vi "CRYCurve Library.vi"() -> ()   [LabVIEW 2013]
uses:
  <vilib>/Utility/miscctls.llb/LVPoint32TypeDef.ctl
  <vilib>/Utility/miscctls.llb/LVBoundsTypeDef.ctl
  <vilib>/Utility/inputDevices.llb/closeMouse.vi
  Global/CRYCurve Library Global.vi
  <vilib>/Utility/inputDevices.llb/mouseAcquire.vi
panel:
  out "StepNameChange":i32
  in  "DragStartFlag":bool
  out "Drop?":bool
  out "AllDragTags":string[](array[string])
  in  "GroupFlag":bool
  out "AllParents":string[](array[string])
  out "Select Row":i32
  out "GroupRowNumber":i32
  out "TreeValue":string[](array[string])
  out "Menu Coords":T1
  in  "Legend":i32(listbox)
  out "OldPos":T2
  out "Coords":T1
  in  "StateOut":bool
  in  "stop":bool
  in  "UndoAutoProtect":bool
  in  "AutoProtect":bool
  in  "CompleteDelete":bool
  in  "Protect":bool
  in  "Delete":bool
  in  "Save":bool
  in  "Open":bool
  out "BottomBar":bool
  in  "CurveLibrary Tab":enum32{"Curves", "Values", "Results", "WFM"}(tab)
  in  "Curves Tree":string[](tree)
  in  "Values Tree":string[](tree)
  in  "Results Tree":string[](tree)
  in  "WFM Tree":string[](tree)
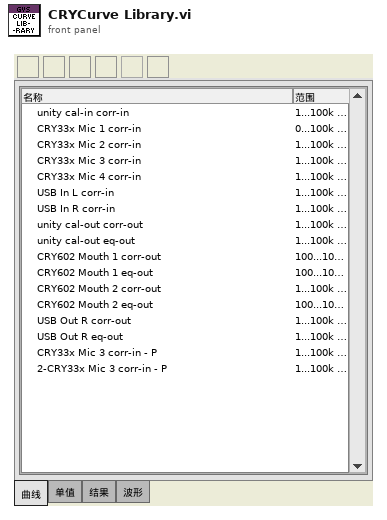
[diagram p1: front panel]
types:
  T1 = typedef "LVPoint32TypeDef.ctl" = cluster{"Horizontal":i32, "Vertical":i32}
  T2 = typedef "LVBoundsTypeDef.ctl" = cluster{"Width":u32, "Height":u32}
  T3 = typedef "CRYCurveLib Info Cluster.ctl" = cluster{"GroupingState":string}
  T4 = cluster{"Horizontal":i32, "Vertical":i32, "Scrolling":i32}
  T5 = cluster{"Shift":bool, "Ctrl":bool, "Alt":bool, "Cmd":bool, "Opt":bool}
  T6 = cluster{"data name":string, "drag data":variant}[]
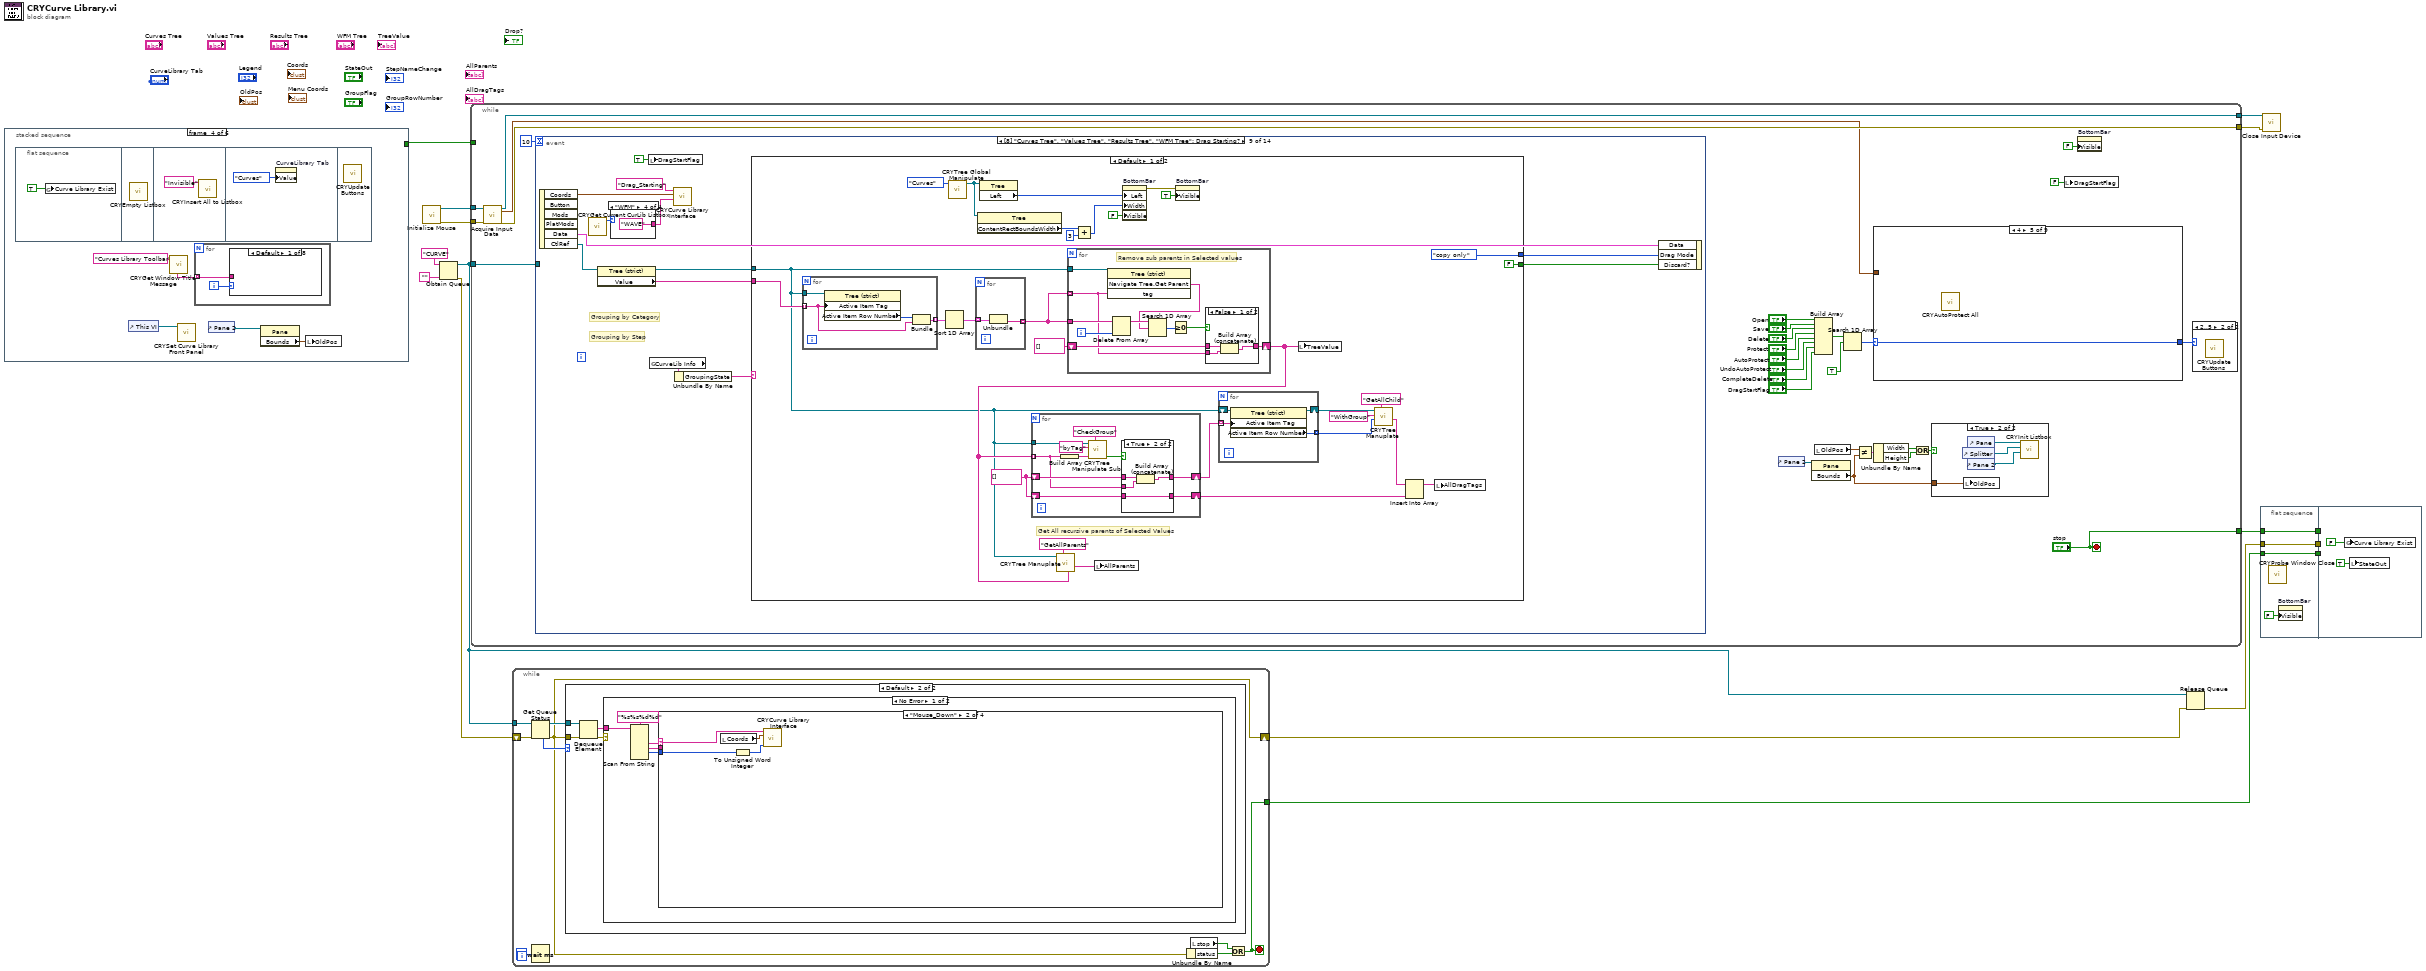
[diagram p0: block diagram]
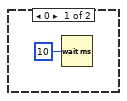
[diagram p2: hidden frame]
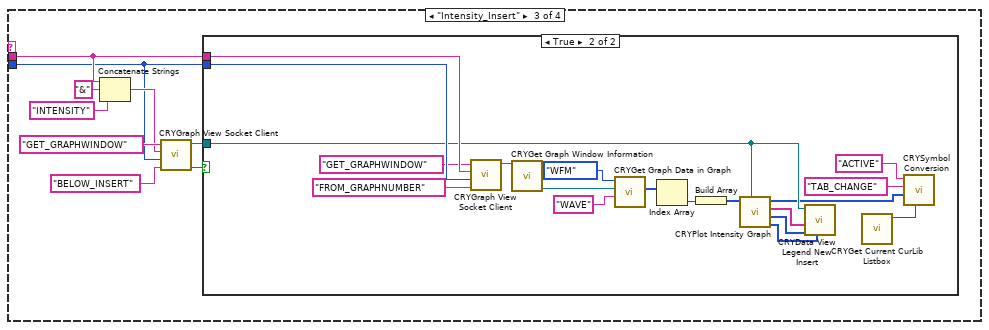
[diagram p4: hidden frame]
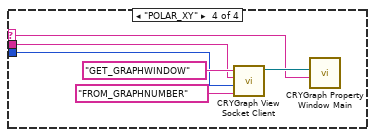
[diagram p6: hidden frame]
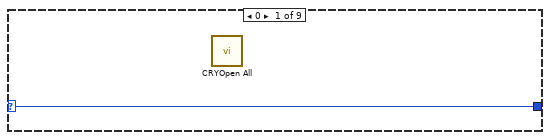
[diagram p10: hidden frame]
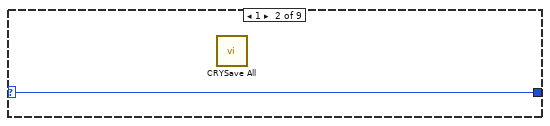
[diagram p11: hidden frame]
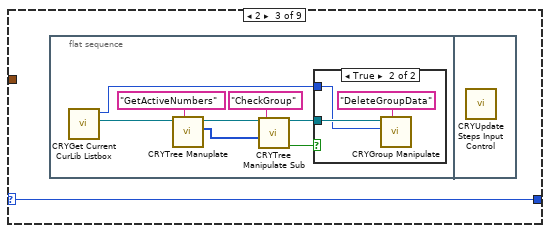
[diagram p12: hidden frame]
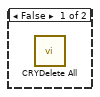
[diagram p13: hidden frame]
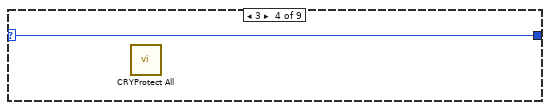
[diagram p14: hidden frame]
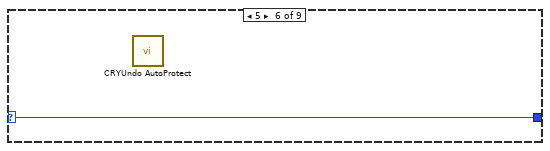
[diagram p15: hidden frame]
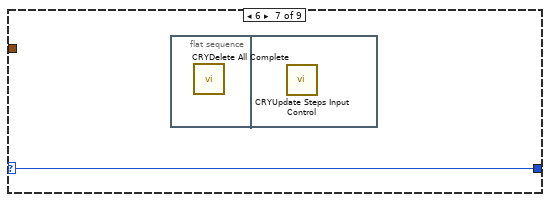
[diagram p16: hidden frame]
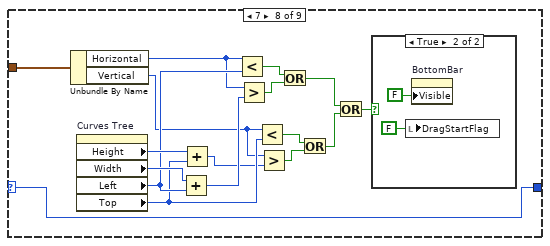
[diagram p17: hidden frame]
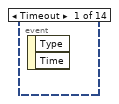
[diagram p20: hidden frame]
diagram:
  n1 = stacked-sequence {
    tunnel: [_ _ _ _ _ w68] -> w13
    frame #0 {
      n2 = control-ref of="Curves Tree"() -> (w19:refnum<vi>)
      n3 = control-ref of="Values Tree"() -> (w18:refnum<vi>)
      n4 = control-ref of="Results Tree"() -> (w17:refnum<vi>)
      n5 = control-ref of="WFM Tree"() -> (w28:refnum<vi>)
      n6 = control-ref of="CurveLibrary Tab"() -> (w27:refnum<vi>)
      n7 = control-ref of="Open"() -> (w26:refnum<vi>)
      n8 = control-ref of="Save"() -> (w25:refnum<vi>)
      n9 = control-ref of="Delete"() -> (w24:refnum<vi>)
      n10 = control-ref of="Protect"() -> (w23:refnum<vi>)
      n11 = control-ref of="AutoProtect"() -> (w22:refnum<vi>)
      n12 = control-ref of="UndoAutoProtect"() -> (w21:refnum<vi>)
      n13 = control-ref of="This VI"() -> (w20:refnum<vi>)
      n14 = global write "CRYCurve Library Global.vi" "Curve Library VI"(w20) -> ()
      n15 = global write "CRYCurve Library Global.vi" "Curves Tree"(w19) -> ()
      n16 = global write "CRYCurve Library Global.vi" "Values Tree"(w18) -> ()
      n17 = global write "CRYCurve Library Global.vi" "Results Tree"(w17) -> ()
      n18 = global write "CRYCurve Library Global.vi" "WFM Tree"(w28) -> ()
      n19 = global write "CRYCurve Library Global.vi" "Curve Library Tab"(w27) -> ()
      n20 = global write "CRYCurve Library Global.vi" "Open Button"(w26) -> ()
      n21 = global write "CRYCurve Library Global.vi" "Save Button"(w25) -> ()
      n22 = global write "CRYCurve Library Global.vi" "Delete Button"(w24) -> ()
      n23 = global write "CRYCurve Library Global.vi" "Protect Button"(w23) -> ()
      n24 = global write "CRYCurve Library Global.vi" "AutoProtect Button"(w22) -> ()
      n25 = global write "CRYCurve Library Global.vi" "UndoAutoProtect Button"(w21) -> ()
      n26 = local write "stop"(FALSE ("stop")) -> ()
    }
    frame #1 {
      n27 = while {
        tunnel: [w31] -> w30
        stop <- w31 stop-if-true
        n28 = global read "CRYCurve Library Global.vi" "Curve Library Global Inserting"() -> (w32:bool)
        n29 = Wait Until Next ms Multiple(millisecond multiple=u32 10 ("milliseconds to wait")) -> ()  [unwired: 1 out]
        n30 = Not(x=w32) -> (.not. x?=w31:bool)
      }
      n31 = global write "CRYCurve Library Global.vi" "Curve Library Loading"(w30) -> ()
    }
    frame #2 {
      n32 = control-ref of="Splitter"() -> (w35:refnum<vi>)
      n33 = control-ref of="Pane"() -> (w36:refnum<vi>)
      n34 = control-ref of="Pane 2"() -> (w34:refnum<vi>)
      n35 = call "CRYInit Listbox.vi"("Pane 2"=w34, "Splitter"=w35, "Pane 1"=w36) -> ()  [unwired: 9 out]
    }
    frame #3 {
      n36 = flat-sequence {
        frame #0 {
          n37 = global write "CRYCurve Library Global.vi" "Curve Library Exist"(TRUE ("Exist")) -> ()
        }
        frame #1 {
          n38 = call "CRYEmpty Listbox.vi"() -> ()  [unwired: 1 out]
        }
        frame #2 {
          n39 = call "CRYInsert All to Listbox.vi"("sAction"="Invisible") -> ()  [unwired: 11 out]
        }
        frame #3 {
          n40 = property on="CurveLibrary Tab" class="TabCtl (strict)"("Value"=enum32{"Curves", "Values", "Results", "WFM"}."Curves" ("Curve Library Tab")) -> ()  [unwired: 2 in, 2 out]
        }
        frame #4 {
          n41 = call "CRYUpdate Buttons.vi"() -> ()  [unwired: 1 in, 11 out]
        }
      }
      n42 = control-ref of="This VI"() -> (w37:refnum<vi>)
      n43 = call "CRYGet Window Title Message.vi"("Kind"="Curves Library Toolbar") -> ("Tip Strip"=w40:string[])  [unwired: 5 in, 5 out]
      n44 = call "CRYSet Curve Library Front Panel.vi"("Vi Ref In"=w37) -> ()  [unwired: 10 in, 1 out]
      n45 = for {
        tunnel: w40 -> [w42] mode=indexing
        i -> [w43]
        n46 = case shown="Default" w43 {
          tunnel: w42 -> [_ w44 w45 w46 w47 w48 w49 w50]
          frame Default {
          }
          frame 0 {
            n47 = property on="Open" class="Bool"("TipStrip"=w44) -> ()  [unwired: 2 in, 2 out]
          }
          frame 1 {
            n48 = property on="Save" class="Bool"("TipStrip"=w45) -> ()  [unwired: 2 in, 2 out]
          }
          frame 2 {
            n49 = property on="Delete" class="Bool"("TipStrip"=w46) -> ()  [unwired: 2 in, 2 out]
          }
          frame 3 {
            n50 = property on="Protect" class="Bool"("TipStrip"=w47) -> ()  [unwired: 2 in, 2 out]
          }
          frame 4 {
            n51 = property on="AutoProtect" class="Bool"("TipStrip"=w48) -> ()  [unwired: 2 in, 2 out]
          }
          frame 5 {
            n52 = property on="UndoAutoProtect" class="Bool"("TipStrip"=w49) -> ()  [unwired: 2 in, 2 out]
          }
          frame 6 {
            n53 = property on="CompleteDelete" class="Bool"("TipStrip"=w50) -> ()  [unwired: 2 in, 2 out]
          }
        }
      }
      n54 = control-ref of="Pane 2"() -> (w38:refnum<vi>)
      n55 = property class="Pane"(reference=w38) -> ("Bounds"=w39:T2)  [unwired: 1 in, 2 out]
      n56 = local write "OldPos"(w39) -> ()
    }
    frame #4 {
      n57 = flat-sequence {
        frame #0 {
          n58 = call "CRYGroup Manipulate.vi"("sAction"="GroupingOff", "sOption"="Invisible") -> ()  [unwired: 6 in, 4 out]
        }
        frame #1 {
          n59 = global read "CRYCurve Library Global.vi" "CurveLib Info"() -> (w57:T3)
          n60 = Unbundle By Name(w57) -> ("GroupingState"=w56:string)
          n61 = case shown="\"Grouping by Category\"" w56 {
            frame "Grouping Off", Default {
              n62 = call "CRYTree Global Manipulate.vi"("sOption"="All") -> ("WFM Tree"=w59:refnum<vi>, "Results Tree"=w60:refnum<vi>, "Values Tree"=w61:refnum<vi>, "Tree/Curve Tree"=w62:refnum<vi>)  [unwired: 7 in]
              n63 = Build Array(w62, w61, w60, w59) -> (w58:refnum<vi>[])
              n64 = for {
                tunnel: w58 -> [w65] mode=indexing
                n65 = property class="Tree"(reference=w65, "Visible"=TRUE) -> ()  [unwired: 1 in, 2 out]
              }
            }
            frame "Grouping by Category" {
              n66 = call "CRYGroup Manipulate.vi"("sAction"="GroupingbyCategory") -> ()  [unwired: 7 in, 4 out]
            }
            frame "Grouping by Step" {
              n67 = call "CRYGroup Manipulate.vi"("sAction"="GroupingbyStep") -> ()  [unwired: 7 in, 4 out]
            }
          }
        }
      }
    }
    frame #5 {
      w68 = FALSE ("Curve Library Loading")
      n68 = call "CRYTree Global Manipulate.vi"("Type In"=enum16{"Curves", "Values", "Results", "WFM"}."Curves") -> ("Tree/Curve Tree"=w73:refnum<vi>)  [unwired: 7 in, 3 out]
      n69 = property class="Tree"(reference=w73) -> ("ContentRectBoundsWidth"=w70:i32)  [unwired: 1 in, 2 out]
      n70 = property class="Tree"(reference=w73) -> ("Left"=w76:i32)  [unwired: 1 in, 2 out]
      n71 = global write "CRYCurve Library Global.vi" "Curve Library Loading"(w68) -> ()
      n72 = local write "DragStartFlag"(w68) -> ()
      n73 = local write "GroupRowNumber"(-1 ("GroupRowNumber")) -> ()
      n74 = Add(x=w70, y=3) -> (x+y=w69:i32)
      n75 = local write "StateOut"(TRUE ("StateOut")) -> ()
      n76 = property on="BottomBar" class="Bool (strict)"("Left"=w76, "Width"=w69, "Visible"=FALSE) -> ()  [unwired: 2 in, 2 out]
    }
  }
  n77 = call <vilib>:"Initialize Mouse.vi"() -> ("error out"=w3:errorcluster, "device ID"=w4:refnum<k1>)  [unwired: 10 in]
  n78 = Obtain Queue(name (unnamed)="CURVE" ("YAxisTitle"), element data type="" ("Action Type")) -> (queue out=w7:refnum<queue>, error out=w6:errorcluster)  [unwired: 3 in, 1 out]
  n79 = while {
    tunnel: w13 -> [_]
    tunnel: ["stop"] -> w12
    tunnel: w7 -> [w101]
    tunnel: w4 -> [w88]
    tunnel: w3 -> [w87]
    tunnel: [w86] -> w2
    tunnel: [w85] -> w1
    stop <- "stop" stop-if-true
    n80 = call-poly <vilib>:"Acquire Input Data.vi"("device ID"=w88, "error in (no error)"=w87) -> ("device ID"=w86:refnum<k1>, "axis info"=w82:T4, "error out"=w85:errorcluster)  [unwired: 14 in, 1 out]
    n81 = event shown="[8] \"Curves Tree\", \"Values Tree\", \"Results Tree\", \"WFM Tree\": Drag Starting?" {
      selector: _ -> [_ _ _ _ _ _ _ _ _ _ _ _ _ _]
      dyn-events: _ -> [_ _ _ _ _ _ _ _ _ _ _ _ _ _]
      timeout: 10 -> [_ _ _ _ _ _ _ _ _ _ _ _ _ _]
      tunnel: w101 -> [_ _ _ _ _ w170 _ _ _ _ _ _ _ _]
      event Timeout {
        n82 = event-data() -> ()  [unwired: 3 out]
      }
      event "CurveLibrary Tab": Value Change {
        n83 = event-data() -> ("NewVal"=w150:enum32{"Curves", "Values", "Results", "WFM"})  [unwired: 6 out]
        n84 = local write "GroupRowNumber"(-1 ("GroupRowNumber")) -> ()
        n85 = call "CRYCurve Library Interface.vi"("nButton"=w150, "sEventName"="Tab_Value_Change") -> ()  [unwired: 9 in, 1 out]
      }
      event Pane Size {
        n86 = event-data() -> ()  [unwired: 7 out]
        n87 = control-ref of="Splitter"() -> (w153:refnum<vi>)
        n88 = call "CRYTree Global Manipulate.vi"("Type In"=enum16{"Curves", "Values", "Results", "WFM"}."Curves") -> ("Tree/Curve Tree"=w159:refnum<vi>)  [unwired: 7 in, 3 out]
        n89 = control-ref of="Pane"() -> (w154:refnum<vi>)
        n90 = control-ref of="Pane 2"() -> (w152:refnum<vi>)
        n91 = property class="Tree"(reference=w159) -> ("ContentRectBoundsWidth"=w155:i32)  [unwired: 1 in, 2 out]
        n92 = call "CRYInit Listbox.vi"("Pane 2"=w152, "Splitter"=w153, "Pane 1"=w154) -> ()  [unwired: 9 in]
        n93 = Add(x=w155, y=3) -> (x+y=w157:i32)
        n94 = property on="BottomBar" class="Bool (strict)"("Width"=w157) -> ()  [unwired: 2 in, 2 out]
      }
      event "Curves Tree", "Values Tree", "Results Tree", "WFM Tree": Shortcut Menu Activation? {
        n95 = event-data() -> ("MenuRef"=w162:refnum<k9>, "Coords"=w161:T1)  [unwired: 1 out]
        n96 = local write "Menu Coords"(w161) -> ()
        n97 = call "CRYCurve Library Interface.vi"("MenuRef"=w162, "Coords"=w161, "sEventName"="Shortcut_Menu_Activation") -> ("bResult"=w160:bool)  [unwired: 8 in]
        n98 = event-data("Discard?"=w160) -> ()  [unwired: 1 in, 1 out]
      }
      event "Curves Tree", "Values Tree", "Results Tree", "WFM Tree": Shortcut Menu Selection (User) {
        n99 = event-data() -> ("ItemTag"=w165:string)  [unwired: 2 out]
        n100 = local read "Menu Coords"() -> (w164:T1)
        n101 = call "CRYCurve Library Interface.vi"("sData"=w165, "Coords"=w164, "sEventName"="Shortcut_Menu_Selection") -> ()  [unwired: 8 in, 1 out]
      }
      event "Curves Tree", "Values Tree", "Results Tree", "WFM Tree": Mouse Down {
        n102 = event-data() -> ("Coords"=w169:T1, "Button"=w168:u16)  [unwired: 2 out]
        n103 = flat-sequence {
          tunnel: w169 -> [w172]
          tunnel: w168 -> [w173]
          tunnel: [w173] -> w171
          tunnel: [w172] -> w167
          tunnel: w171 -> [w177]
          tunnel: w170 -> [_]
          tunnel: w167 -> [w176]
          frame #0 {
            n104 = To Unsigned Word Integer(number=w173) -> (unsigned 16bit integer=w175:u16)
            n105 = call "CRYCurve Library Interface.vi"("nButton"=w175, "Coords"=w172, "sEventName"="Mouse_Down_Right") -> ()  [unwired: 8 in, 1 out]
          }
          frame #1 {
            n106 = call "CRYCurve Library Interface.vi"("nButton"=w177, "Coords"=w176, "sEventName"="Mouse_Down") -> ()  [unwired: 8 in, 1 out]
          }
        }
      }
      event "Curves Tree", "Values Tree", "Results Tree", "WFM Tree": Key Down {
        n107 = event-data() -> ("ScanCode"=w180:i16, "PlatMods"=w179:T5)  [unwired: 2 out]
        n108 = call "CRYCurve Library Interface.vi"("PlatMods"=w179, "nButton"=w180, "sEventName"="Key_Down") -> ()  [unwired: 8 in, 1 out]
      }
      event "Curves Tree", "Values Tree", "Results Tree", "WFM Tree": Double Click {
        n109 = event-data() -> ("Coords"=w182:T1)  [unwired: 5 out]
        n110 = call "CRYCurve Library Interface.vi"("Coords"=w182, "sEventName"="Double_Click") -> ()  [unwired: 9 in, 1 out]
      }
      event "Curves Tree", "Values Tree", "Results Tree", "WFM Tree": Drag Starting? {
        # "Grouping by Step"
        # "Grouping by Category"
        n111 = event-data() -> ("Coords"=w195:T1, "Data"=w191:T6, "CtlRef"=w190:refnum<vi>)  [unwired: 4 out]
        n112 = call "CRYGet Current CurLib Listbox.vi"() -> ("Type"=w193:enum16{"Curves", "Values", "Results", "WFM"})  [unwired: 9 in, 2 out]
        n113 = property class="Tree (strict)"(reference=w190) -> (reference out=w188:refnum<vi>, "Value"=w189:string[])  [unwired: 1 in, 1 out]
        n114 = case shown="\"WFM\"" w193 {
          tunnel: ["XY" ("GraphType") "TABLE" ("GraphType") "RESULT" ("GraphType") "WAVE" ("GraphType")] -> w192
          frame "Curves", Default {
          }
          frame "Values" {
          }
          frame "Results" {
          }
          frame "WFM" {
          }
        }
        n115 = local write "DragStartFlag"(TRUE ("DragStartFlag")) -> ()
        n116 = global read "CRYCurve Library Global.vi" "CurveLib Info"() -> (w186:T3)
        n117 = call "CRYCurve Library Interface.vi"("sData"=w192, "Coords"=w195, "sEventName"="Drag_Starting") -> ()  [unwired: 8 in, 1 out]
        n118 = Unbundle By Name(w186) -> ("GroupingState"=w185:string)
        n119 = case shown="Default" w185 {
          tunnel: [enum32{"copy or move", "copy only", "move only"}."copy only" ("Drag Mode") enum32{"copy or move", "copy only", "move only"}."copy only" ("Drag Mode")] -> w196
          tunnel: w189 -> [w223 _]
          tunnel: w188 -> [w211 _]
          tunnel: [FALSE ("Discard?") TRUE ("Discard?")] -> w184
          frame Default {
            w215 = string[] []
            # "Get All recursive parents of Selected Values"
            n120 = for {
              tunnel: w223 -> [w265] mode=indexing
              tunnel: w211 -> [w267]
              tunnel: [w264] -> w222 mode=indexing
              n121 = property class="Tree (strict)"(reference=w267, "Active Item Tag"=w265) -> ("Active Item Row Number"=w266:i32)  [unwired: 1 in, 2 out]
              n122 = Bundle("Active Item Row Number"=w266, w265) -> (w264:cluster{"Active Item Row Number":i32, string})  [unwired: 1 in]
            }
            n123 = Sort 1D Array(array=w222) -> (sorted array=w221:cluster{"Active Item Row Number":i32, string}[])
            n124 = call "CRYTree Global Manipulate.vi"("Type In"=enum16{"Curves", "Values", "Results", "WFM"}."Curves") -> ("Tree/Curve Tree"=w201:refnum<vi>)  [unwired: 7 in, 3 out]
            n125 = for {
              tunnel: w221 -> [w263] mode=indexing
              tunnel: [w262] -> w220 mode=indexing
              n126 = Unbundle(w263) -> (w262:string)  [unwired: 1 out]
            }
            n127 = property class="Tree"(reference=w201) -> ("ContentRectBoundsWidth"=w204:i32)  [unwired: 1 in, 2 out]
            n128 = property class="Tree"(reference=w201) -> ("Left"=w199:i32)  [unwired: 1 in, 2 out]
            n129 = for {
              tunnel: w220 -> [w248] mode=indexing
              tunnel: w211 -> [w257]
              tunnel: w220 -> [w251]
              shift-right: [w253] -> w217
              shift-left: string[] [] -> [w254]
              i -> [w252]
              # "Remove sub parents in Selected values"
              n130 = invoke class="Tree (strict)" method="Navigate Tree.Get Parent"(reference=w257, "tag"=w248) -> ("Navigate Tree:Get Parent"=w249:string)  [unwired: 2 in, 3 out]
              n131 = Delete From Array(array=w251, index=w252) -> (array with subset deleted=w250:string[])  [unwired: 1 in, 1 out]
              n132 = Search 1D Array(1D array=w250, element=w249) -> (index of element=w256:i32)  [unwired: 1 in]
              n133 = Greater Or Equal To 0?(x=w256) -> (x >= 0?=w255:bool)
              n134 = case shown="False" w255 {
                tunnel: w254 -> [w260 w261]
                tunnel: [w259 w261] -> w253
                tunnel: w248 -> [w258 _]
                frame False {
                  n135 = Build Array (concatenate)(w260, w258) -> (w259:string[])
                }
                frame True {
                }
              }
            }
            n136 = for {
              tunnel: w217 -> [w232] mode=indexing
              tunnel: w211 -> [w235]
              shift-right: [w239] -> w206
              shift-left: w215 -> [w238]
              shift-right: [w230] -> w214
              shift-left: w215 -> [w231]
              n137 = Build Array(w232) -> (w234:string[])
              n138 = call "CRYTree Manipulate Sub.vi"("sAction"="CheckGroup", "sData"=w234, "sOption"="byTag", "Tree in"=w235) -> ("bData out"=w233:bool)  [unwired: 3 in, 4 out]
              n139 = case shown="True" w233 {
                tunnel: w238 -> [w243 w247]
                tunnel: [w243 w246] -> w239
                tunnel: w232 -> [w241 w245]
                tunnel: w231 -> [w242 w244]
                tunnel: [w240 w244] -> w230
                frame False {
                  n140 = Build Array (concatenate)(w242, w241) -> (w240:string[])
                }
                frame True {
                  n141 = Build Array (concatenate)(w247, w245) -> (w246:string[])
                }
              }
            }
            n142 = call "CRYTree Manuplate.vi"("sData"=w217, "sAction"="GetAllParents", "Tree in"=w211) -> ("sData Out"=w216:string[])  [unwired: 5 in, 3 out]
            n143 = Add(x=w204, y=3) -> (x+y=w205:i32)
            n144 = local write "AllParents"(w216) -> ()
            n145 = property on="BottomBar" class="Bool (strict)"("Left"=w199, "Width"=w205, "Visible"=FALSE) -> (error out=w198:errorcluster)  [unwired: 2 in, 1 out]
            n146 = property on="BottomBar" class="Bool (strict)"(error in=w198, "Visible"=TRUE) -> ()  [unwired: 1 in, 2 out]
            n147 = for {
              tunnel: w206 -> [w228] mode=indexing
              tunnel: [w227] -> w209 mode=indexing
              shift-right: [w226] -> w210
              shift-left: w211 -> [w229]
              n148 = property class="Tree (strict)"(reference=w229, "Active Item Tag"=w228) -> (reference out=w226:refnum<vi>, "Active Item Row Number"=w227:i32)  [unwired: 1 in, 1 out]
            }
            n149 = local write "TreeValue"(w217) -> ()
            n150 = call "CRYTree Manuplate.vi"("sAction"="GetAllChild", "nData"=w209, "sOption"="WithGroup", "Tree in"=w210) -> ("sData Out"=w208:string[])  [unwired: 4 in, 3 out]
            n151 = Insert Into Array(array=w208, new element=w214) -> (w213:string[])  [unwired: 1 in]
            n152 = local write "AllDragTags"(w213) -> ()
          }
          frame "Grouping by Category", "Grouping by Step" {
          }
        }
        n153 = event-data("Data"=w191, "Drag Mode"=w196, "Discard?"=w184) -> ()  [unwired: 1 in, 1 out]
      }
      event "Curves Tree", "Values Tree", "Results Tree", "WFM Tree": event type 3.0.xa000003a {
        n154 = event-data() -> ("CtlRef"=w281:refnum<vi>, "Coords"=w309:T1)  [unwired: 8 out]
        n155 = Unbundle By Name(w309) -> ("Horizontal"=w293:i32, "Vertical"=w318:i32)
        n156 = local read "TreeValue"() -> (w280:string[])
        n157 = local read "AllDragTags"() -> (w279:string[])
        n158 = call "CRYGet Tree Click State.vi"("Coords"=w309, "Tree Ref In"=w281) -> ("Row Number"=w306:i32, "Tag"=w275:string)  [unwired: 4 in, 4 out]
        n159 = for {
          tunnel: w281 -> [w411]
          tunnel: w280 -> [w410] mode=indexing
          tunnel: [w409] -> w334 mode=indexing
          n160 = property class="Tree (strict)"(reference=w411, "Active Item Tag"=w410) -> ("Active Item Row Number"=w409:i32)  [unwired: 1 in, 2 out]
        }
        n161 = case shown="0, Default" w306 {
          selector: w306 -> [w374 _]
          tunnel: w281 -> [w378 w380]
          tunnel: [w376 w380] -> w308
          tunnel: [w375 FALSE ("bData out")] -> w327
          frame 0, Default {
            n162 = Build Array(w374) -> (w377:i32[])
            n163 = call "CRYTree Manipulate Sub.vi"("sAction"="CheckGroup", "nData"=w377, "Tree in"=w378) -> ("bData out"=w375:bool, "Tree Out"=w376:refnum<vi>)  [unwired: 4 in, 3 out]
          }
          frame -1 {
          }
        }
        n164 = case shown="True" w327 {
          tunnel: w318 -> [w389 w398]
          tunnel: w281 -> [w385 w406]
          tunnel: w306 -> [w384 w395]
          tunnel: [w383 w393] -> w311
          tunnel: [FALSE w396] -> w326
          frame False {
            n165 = Decrement(x=w384) -> (x-1=w387:i32)
            n166 = property class="Tree (strict)"(reference=w385, "Active Item Row Number"=w384, "ActiveColNum"=0 ("Active Cell:Active Column Number")) -> ("ActiveCellPosTop"=w388:i32)  [unwired: 1 in, 2 out]
            n167 = Add(x=w388, y=6) -> (x+y=w390:i32)
            n168 = Greater Or Equal?(x=w390, y=w389) -> (x >= y?=w386:bool)
            n169 = Select(t=w387, s=w386, f=w384) -> (s? t:f=w383:i32)
          }
          frame True {
            n170 = Decrement(x=w395) -> (x-1=w399:i32)
            n171 = property class="Tree (strict)"(reference=w406, "Active Item Row Number"=w395, "ActiveColNum"=0 ("Active Cell:Active Column Number")) -> ("ActiveCellPosTop"=w403:i32)  [unwired: 1 in, 2 out]
            n172 = Add(x=w403, y=4) -> (x+y=w397:i32)
            n173 = Add(x=w403, y=12) -> (x+y=w405:i32)
            n174 = Less Or Equal?(x=w398, y=w397) -> (x <= y?=w402:bool)
            n175 = Greater Or Equal?(x=w398, y=w405) -> (x >= y?=w401:bool)
            n176 = Compound Arithmetic op=AND(invert w401, invert w402) -> (w396:bool)
            n177 = Compound Arithmetic op=AND(w401, invert w396) -> (w400:bool)
            n178 = Select(t=w395, s=w400, f=w399) -> (s? t:f=w394:i32)
            n179 = Select(t=w395, s=w396, f=w394) -> (s? t:f=w393:i32)
          }
        }
        n180 = Array Size(array=w334) -> (size(s)=w333:i32)
        n181 = Sort 1D Array(array=w334) -> (sorted array=w332:i32[])
        n182 = Decrement(x=w333) -> (x-1=w331:i32)
        n183 = Index Array(array=w332, index=w331) -> (element=w330:i32)
        n184 = Equal?(x=w311, y=w330) -> (x = y?=w329:bool)
        n185 = property class="Tree (strict)"(reference=w281) -> ("ContentRectPosLeft"=w298:i32, "ContentRectBoundsWidth"=w294:i32)  [unwired: 1 in, 2 out]
        n186 = property class="Tree (strict)"(reference=w281) -> (reference out=w288:refnum<vi>, "All Tags"=w301:string[], "ContentRectPosTop"=w299:i32, "DispItems"=w290:string[])  [unwired: 1 in, 1 out]
        n187 = Greater Or Equal?(x=w311, y=-1) -> (x >= y?=w307:bool)
        n188 = Array Size(array=w301) -> (size(s)=w300:i32)
        n189 = Array Size(array=w290) -> (size(s)=w312:i32)
        n190 = Add(x=w298, y=w294) -> (x+y=w297:i32)
        n191 = Decrement(x=w300) -> (x-1=w313:i32)
        n192 = Multiply(x=w312, y=16) -> (x*y=w314:i32)
        n193 = Less Or Equal?(x=w293, y=w298) -> (x <= y?=w296:bool)
        n194 = Greater Or Equal?(x=w293, y=w297) -> (x >= y?=w295:bool)
        n195 = Compound Arithmetic op=OR(w296, w295) -> (w292:bool)
        n196 = Add(x=w299, y=w314) -> (x+y=w317:i32)
        n197 = Add(x=w299, y=16) -> (x+y=w321:i32)
        n198 = Less Than 0?(x=w311) -> (x < 0?=w324:bool)
        n199 = Less Or Equal?(x=w318, y=w321) -> (x <= y?=w325:bool)
        n200 = Greater Or Equal?(x=w318, y=w317) -> (x >= y?=w316:bool)
        n201 = Compound Arithmetic op=AND(w325, w324) -> (w323:bool)
        n202 = Select(t=-1, s=w323, f=w311) -> (s? t:f=w315:i32)
        n203 = Select(t=w313, s=w316, f=w315) -> (s? t:f=w286:i32)
        n204 = property class="Tree (strict)"(reference=w281, "Active Item Row Number"=w286, "ActiveColNum"=0 ("Active Cell:Active Column Number")) -> ("ActiveCellPosTop"=w304:i32)  [unwired: 1 in, 2 out]
        n205 = Add(x=w304, y=12) -> (x+y=w303:i32)
        n206 = Equal?(x=-1 ("y"), y=w286) -> (x = y?=w283:bool)
        n207 = property class="Tree (strict)"(reference=w281, "Active Item Row Number"=w286) -> (reference out=w277:refnum<vi>, "Active Item Tag"=w287:string)  [unwired: 1 in, 1 out]
        n208 = Search 1D Array(1D array=w290, element=w287) -> (index of element=w289:i32)  [unwired: 1 in]
        n209 = Greater Or Equal To 0?(x=w289) -> (x >= 0?=w284:bool)
        n210 = Compound Arithmetic op=OR(w284, w283) -> (w282:bool)
        n211 = case shown="False" w282 {
          tunnel: w288 -> [w337 _]
          tunnel: [w338 w340] -> w276
          tunnel: w286 -> [_ w340]
          tunnel: w287 -> [w336 _]
          frame False {
            n212 = invoke class="Tree (strict)" method="Navigate Tree.Get Parent"(reference=w337, "tag"=w336) -> ("Navigate Tree:Get Parent"=w339:string)  [unwired: 2 in, 3 out]
            n213 = property class="Tree (strict)"(reference=w337, "Active Item Tag"=w339) -> ("Active Item Row Number"=w338:i32)  [unwired: 1 in, 2 out]
          }
          frame True {
          }
        }
        "Select Row" <- w276
        n214 = property class="Tree (strict)"(reference=w277, "Active Item Row Number"=w276) -> ("Active Item Tag"=w274:string)  [unwired: 1 in, 2 out]
        n215 = Search 1D Array(1D array=w279, element=w274) -> (index of element=w335:i32)  [unwired: 1 in]
        n216 = Less Than 0?(x=w335) -> (x < 0?=w328:bool)
        n217 = Compound Arithmetic op=AND(invert w292, invert w329, w328) -> (w278:bool)
        n218 = Compound Arithmetic op=AND(w278, w327, w326) -> (w291:bool)
        n219 = local write "GroupFlag"(w291) -> ()
        n220 = case shown="False" w291 {
          tunnel: w275 -> [_ w368]
          tunnel: w308 -> [w342 w373]
          tunnel: w306 -> [_ w366]
          tunnel: w307 -> [w345 _]
          tunnel: w278 -> [w344 _]
          tunnel: w303 -> [w343 _]
          frame False {
            n221 = local read "GroupRowNumber"() -> (w341:i32)
            n222 = case shown="True" w345 {
              tunnel: w343 -> [_ w358]
              tunnel: w344 -> [_ w356]
              frame False {
              }
              frame True {
                n223 = property on="BottomBar" class="Bool (strict)"() -> ("Visible"=w357:bool)  [unwired: 2 in, 2 out]
                n224 = case shown="False" w357 {
                  tunnel: w358 -> [w361 w364]
                  tunnel: w356 -> [w360 w363]
                  frame False {
                    n225 = property on="BottomBar" class="Bool (strict)"("Top"=w361) -> (error out=w359:errorcluster)  [unwired: 2 in, 1 out]
                    n226 = property on="BottomBar" class="Bool (strict)"(error in=w359, "Visible"=w360) -> ()  [unwired: 1 in, 2 out]
                  }
                  frame True {
                    n227 = property on="BottomBar" class="Bool (strict)"("Visible"=w363) -> (error out=w362:errorcluster)  [unwired: 2 in, 1 out]
                    n228 = property on="BottomBar" class="Bool (strict)"(error in=w362, "Top"=w364) -> ()  [unwired: 1 in, 2 out]
                  }
                }
              }
            }
            n229 = case shown="0, Default" w341 {
              selector: w341 -> [w346 _]
              tunnel: w342 -> [w355 _]
              frame 0, Default {
                n230 = property class="Tree"(reference=w355) -> (reference out=w354:refnum<vi>, "Value"=w353:variant)  [unwired: 1 in, 1 out]
                n231 = property class="Tree"(reference=w355, "Active Item Row Number"=w346) -> ("Active Item Tag"=w351:string)  [unwired: 1 in, 2 out]
                n232 = Variant To Data(type=string[] [] ("TreeValue"), Variant=w353) -> (data=w350:string[])  [unwired: 1 in, 1 out]
                n233 = Search 1D Array(1D array=w350, element=w351) -> (index of element=w349:i32)  [unwired: 1 in]
                n234 = Delete From Array(array=w350, length=1, index=w349) -> (array with subset deleted=w347:string[])  [unwired: 1 out]
                n235 = property class="Tree"(reference=w354, "Value"=w347) -> ()  [unwired: 1 in, 2 out]
              }
              frame -1 {
              }
            }
          }
          frame True {
            n236 = property class="Tree"(reference=w373) -> (reference out=w372:refnum<vi>, "Value"=w371:variant)  [unwired: 1 in, 1 out]
            n237 = local write "GroupRowNumber"(w366) -> ()
            n238 = property on="BottomBar" class="Bool (strict)"("Visible"=FALSE) -> ()  [unwired: 2 in, 2 out]
            n239 = Variant To Data(type=string[] [] ("TreeValue"), Variant=w371) -> (data=w369:string[])  [unwired: 1 in, 1 out]
            n240 = Build Array (concatenate)(w369, w368) -> (w367:string[])
            n241 = property class="Tree"(reference=w372, "Value"=w367) -> ()  [unwired: 1 in, 2 out]
          }
        }
        n242 = local write "Drop?"(w278) -> ()
        n243 = event-data("Accepted?"=w278) -> ()  [unwired: 1 in, 1 out]
      }
      event "Curves Tree", "Values Tree", "Results Tree", "WFM Tree", "BottomBar": Drag Enter {
        n244 = event-data() -> ()  [unwired: 10 out]
        n245 = event-data("Accepted?"=TRUE) -> ()  [unwired: 1 in, 1 out]
      }
      event "Curves Tree", "Values Tree", "Results Tree", "WFM Tree": Drop {
        n246 = event-data() -> ("CtlRef"=w416:refnum<vi>)  [unwired: 9 out]
        n247 = local read "Drop?"() -> (w415:bool)
        n248 = local write "DragStartFlag"(FALSE ("DragStartFlag")) -> ()
        n249 = property on="BottomBar" class="Bool (strict)"("Visible"=FALSE) -> ()  [unwired: 2 in, 2 out]
        n250 = case shown="True" w415 {
          tunnel: w416 -> [_ w428]
          frame False {
          }
          frame True {
            w440 = string[] []
            n251 = local read "Select Row"() -> (w432:i32)
            n252 = Less Than 0?(x=w432) -> (x < 0?=w431:bool)
            n253 = property class="Tree (strict)"(reference=w428, "Active Item Row Number"=w432) -> (reference out=w446:refnum<vi>, "Active Item Tag"=w421:string)  [unwired: 1 in, 1 out]
            n254 = local read "TreeValue"() -> (w435:string[])
            n255 = case shown="False" w431 {
              tunnel: w446 -> [w457 _]
              tunnel: [w460 FALSE ("bData out")] -> w419
              tunnel: w421 -> [w455 _]
              tunnel: [w462 ""] -> w420
              frame False {
                n256 = Build Array(w455) -> (w464:string[])
                n257 = property class="Tree (strict)"(reference=w457, "Active Item Tag"=w455) -> ("Open?"=w451:bool)  [unwired: 1 in, 2 out]
                n258 = local read "GroupFlag"() -> (w461:bool)
                n259 = Build Array(w455) -> (w456:string[])
                n260 = call "CRYTree Manipulate Sub.vi"("sAction"="CheckGroup", "sData"=w464, "sOption"="byTag", "Tree in"=w457) -> ("bData out"=w450:bool, "Tree Out"=w463:refnum<vi>)  [unwired: 3 in, 3 out]
                n261 = call "CRYTree Manipulate Sub.vi"("sAction"="GetTags", "sData"=w456, "sOption"="Childs" ("sData"), "Tree in"=w457) -> ("sData Out"=w454:string[])  [unwired: 3 in, 4 out]
                n262 = Array Size(array=w454) -> (size(s)=w453:i32)
                n263 = Not Equal To 0?(x=w453) -> (x != 0?=w452:bool)
                n264 = Compound Arithmetic op=AND(w450, w451, w452) -> (w449:bool)
                n265 = Compound Arithmetic op=OR(w461, w449) -> (w460:bool)
                n266 = case shown="True" w460 {
                  tunnel: w455 -> [w469 w470]
                  tunnel: w463 -> [w468 _]
                  tunnel: [w467 w470] -> w462
                  frame False {
                    n267 = invoke class="Tree" method="Navigate Tree.Get Parent"(reference=w468, "tag"=w469) -> ("Navigate Tree:Get Parent"=w467:string)  [unwired: 2 in, 3 out]
                  }
                  frame True {
                  }
                }
              }
              frame True {
                # "In th case of Droppinng in Column Header."
              }
            }
            n268 = for {
              tunnel: w435 -> [w483] mode=indexing
              shift-right: [w489] -> w439
              shift-left: w440 -> [w487]
              shift-right: [w486] -> w434
              shift-left: w440 -> [w484]
              tunnel: w428 -> [w481]
              n269 = Build Array(w483) -> (w490:string[])
              n270 = Build Array (concatenate)(w484, w483) -> (w482:string[])
              n271 = Build Array (concatenate)(w487, w483) -> (w485:string[])
              n272 = call "CRYTree Manipulate Sub.vi"("sAction"="CheckGroup", "sData"=w490, "sOption"="byTag", "Tree in"=w481) -> ("bData out"=w488:bool)  [unwired: 3 in, 4 out]
              n273 = Select(t=w485, s=w488, f=w487) -> (s? t:f=w489:string[])
              n274 = Select(t=w484, s=w488, f=w482) -> (s? t:f=w486:string[])
            }
            n275 = Build Array(w420) -> (w444:string[])
            n276 = for {
              shift-right: [w524] -> w430
              shift-left: w428 -> [w519]
              tunnel: w435 -> [w523] mode=indexing
              tunnel: w420 -> [w521]
              tunnel: w421 -> [w517]
              tunnel: w419 -> [w516]
              shift-right: [w515] -> _
              shift-left: _ -> [w514]
              i -> [w518]
              # "Normally Drop"
              n277 = case shown="False" w516 {
                tunnel: w517 -> [w534 w537]
                tunnel: [w533 w537] -> w520
                tunnel: w519 -> [w535 _]
                tunnel: w521 -> [w533 _]
                tunnel: w518 -> [w526 w536]
                tunnel: [w525 w536] -> w515
                tunnel: w514 -> [_ _]
                frame False {
                  n278 = Build Array(w533) -> (w530:string[])
                  n279 = call "CRYTree Manipulate Sub.vi"("sAction"="GetTags", "sData"=w530, "sOption"="Childs" ("sData"), "Tree in"=w535) -> ("sData Out"=w529:string[])  [unwired: 3 in, 4 out]
                  n280 = Search 1D Array(1D array=w529, element=w534) -> (index of element=w528:i32)  [unwired: 1 in]
                  n281 = Increment(x=w528) -> (x+1=w527:i32)
                  n282 = Add(x=w527, y=w526) -> (x+y=w525:i32)
                }
                frame True {
                }
              }
              n283 = invoke class="Tree (strict)" method="Edit Tree Items.Move Item"(reference=w519, "tag"=w523, "New Parent"=w520, "New Position"=w515, "Carry Children"=TRUE ("Carry Children?")) -> (reference out=w524:refnum<vi>)  [unwired: 2 in, 6 out]
            }
            n284 = Build Array(w420) -> (w422:string[])
            n285 = call "CRYTree Manipulate Sub.vi"("sAction"="GetTags", "sData"=w444, "sOption"="Childs", "Tree in"=w429) -> ("sData Out"=w443:string[], "Tree Out"=w442:refnum<vi>)  [unwired: 3 in, 3 out]
            n286 = local read "AllParents"() -> (w426:string[])
            n287 = for {
              tunnel: w443 -> [w494] mode=indexing
              tunnel: [w497] -> w437
              tunnel: w442 -> [w495]
              i -> [w497]
              stop <- w498 stop-if-true
              n288 = Build Array(w494) -> (w493:string[])
              n289 = call "CRYTree Manipulate Sub.vi"("sAction"="CheckGroup", "sData"=w493, "sOption"="byTag", "Tree in"=w495) -> ("bData out"=w499:bool)  [unwired: 3 in, 4 out]
              n290 = Not(x=w499) -> (.not. x?=w498:bool)
            }
            n291 = for {
              tunnel: w439 -> [w480] mode=indexing
              tunnel: w420 -> [w479]
              tunnel: w437 -> [w478]
              shift-right: [w474] -> w438
              shift-left: w429 -> [w475]
              i -> [w477]
              # "Move Group"
              n292 = Add(x=w478, y=w477) -> (x+y=w476:i32)
              n293 = invoke class="Tree (strict)" method="Edit Tree Items.Move Item"(reference=w475, "tag"=w480, "New Parent"=w479, "New Position"=w476, "Carry Children"=TRUE ("Carry Children?")) -> (reference out=w474:refnum<vi>)  [unwired: 2 in, 6 out]
            }
            n294 = for {
              tunnel: w434 -> [w509] mode=indexing
              tunnel: w420 -> [w512]
              shift-right: [w511] -> w436
              shift-left: w438 -> [w508]
              tunnel: w434 -> [w503]
              i -> [w501]
              # "Move Non-Group data"
              n295 = Array Subset(array=w503, index=w501) -> (w502:string[])  [unwired: 1 in]
              n296 = Build Array (concatenate)(w509, w512, w502) -> (w505:string[])
              n297 = call "CRYTree Manuplate.vi"("sData"=w505, "sAction"="FindInsertLoc", "sOption"="Drop", "Tree in"=w508) -> ("nData Out"=w504:i32[], "Tree Out"=w513:refnum<vi>)  [unwired: 4 in, 2 out]
              n298 = Index Array(array=w504) -> (element=w510:i32)  [unwired: 1 in]
              n299 = invoke class="Tree" method="Edit Tree Items.Move Item"(reference=w513, "tag"=w509, "New Parent"=w512, "New Position"=w510) -> (reference out=w511:refnum<vi>)  [unwired: 3 in, 6 out]
            }
            n300 = flat-sequence {
              tunnel: w430 -> [w447]
              tunnel: [w447] -> w429
              frame #0 {
                # "Visual Effect"
                n301 = Wait (ms)(milliseconds to wait=u32 300) -> ()  [unwired: 1 out]
              }
            }
            n302 = property class="Tree"(reference=w436, "Value"=w435) -> (reference out=w424:refnum<vi>)  [unwired: 1 in, 1 out]
            n303 = call "CRYTree Manuplate.vi"("sData"=w422, "sAction"="GetAllParents", "Tree in"=w424) -> ("sData Out"=w425:string[], "Tree Out"=w423:refnum<vi>)  [unwired: 5 in, 2 out]
            n304 = Build Array (concatenate)(w425, w426) -> (w433:string[])
            n305 = call "CRYGroup Manipulate Sub.vi"("sAction"="MakeGroupName", "sOption"="ChangeNum", "sData"=w433, "Tree in"=w423) -> ()  [unwired: 3 in, 5 out]
          }
        }
        n306 = event-data("Accepted?"=w415) -> ()  [unwired: 1 in, 1 out]
      }
      event "Curves Tree", "Values Tree", "Results Tree", "WFM Tree", "BottomBar": event #0x3d {
        n307 = event-data() -> ()  [unwired: 6 out]
        n308 = local write "DragStartFlag"(FALSE ("DragStartFlag")) -> ()
        n309 = property on="BottomBar" class="Bool (strict)"("Visible"=FALSE) -> ()  [unwired: 2 in, 2 out]
      }
      event "StepNameChange": Value Change {
        n310 = event-data() -> ("NewVal"=w541:i32)  [unwired: 6 out]
        n311 = Build Array(w541) -> (w540:i32[])
        n312 = call "CRYGroup Manipulate.vi"("sAction"="GroupRename", "nData"=w540) -> ()  [unwired: 6 in, 4 out]
      }
    }
    n313 = control-ref of="Pane 2"() -> (w89:refnum<vi>)
    n314 = property class="Pane"(reference=w89) -> ("Bounds"=w90:T2)  [unwired: 1 in, 2 out]
    n315 = Build Array("Open", "Save", "Delete", "Protect", "AutoProtect", "UndoAutoProtect", "CompleteDelete", "DragStartFlag") -> (w105:bool[])
    n316 = local read "OldPos"() -> (w95:T2)
    n317 = Search 1D Array(1D array=w105, element=TRUE) -> (index of element=w103:i32)  [unwired: 1 out]
    n318 = Not Equal?(x=w95, y=w90) -> (x != y?=w94:cluster{"Width":bool, "Height":bool})
    n319 = case shown="4" w103 {
      selector: w103 -> [w111 w112 w113 w125 w126 w127 w128 w145 w148]
      tunnel: [w111 w112 w113 w125 w126 w127 w128 w145 w148] -> w102
      tunnel: w82 -> [_ _ _ _ _ _ _ w129 _]
      frame 0 {
        n320 = call "CRYOpen All.vi"() -> ()  [unwired: 12 out]
      }
      frame 1 {
        n321 = call "CRYSave All.vi"() -> ()  [unwired: 12 out]
      }
      frame 2 {
        n322 = flat-sequence {
          frame #0 {
            n323 = call "CRYGet Current CurLib Listbox.vi"() -> ("CurLib Tree"=w117:refnum<vi>, "Type"=w114:enum16{"Curves", "Values", "Results", "WFM"})  [unwired: 9 in, 1 out]
            n324 = call "CRYTree Manuplate.vi"("sAction"="GetActiveNumbers", "Tree in"=w117) -> ("nData Out"=w121:i32[], "Tree Out"=w120:refnum<vi>)  [unwired: 6 in, 2 out]
            n325 = call "CRYTree Manipulate Sub.vi"("sAction"="CheckGroup", "nData"=w121, "Tree in"=w120) -> ("bData out"=w118:bool, "Tree Out"=w115:refnum<vi>)  [unwired: 4 in, 3 out]
            n326 = case shown="True" w118 {
              tunnel: w115 -> [_ w123]
              tunnel: w114 -> [_ w122]
              frame False {
                n327 = call "CRYDelete All.vi"() -> ()  [unwired: 3 in, 9 out]
              }
              frame True {
                n328 = call "CRYGroup Manipulate.vi"("sAction"="DeleteGroupData", "Type"=w122, "Tree in"=w123) -> ()  [unwired: 5 in, 4 out]
              }
            }
          }
          frame #1 {
            n329 = call "CRYUpdate Steps Input Control.vi"() -> ()  [unwired: 12 in]
          }
        }
      }
      frame 3 {
        n330 = call "CRYProtect All.vi"() -> ()  [unwired: 4 in, 8 out]
      }
      frame 4 {
        n331 = call "CRYAutoProtect All.vi"() -> ()  [unwired: 10 in, 2 out]
      }
      frame 5 {
        n332 = call "CRYUndo AutoProtect.vi"() -> ()  [unwired: 12 out]
      }
      frame 6 {
        n333 = flat-sequence {
          frame #0 {
            n334 = call "CRYDelete All Complete.vi"() -> ()  [unwired: 10 in, 2 out]
          }
          frame #1 {
            n335 = call "CRYUpdate Steps Input Control.vi"() -> ()  [unwired: 12 in]
          }
        }
      }
      frame 7 {
        n336 = Unbundle By Name(w129) -> ("Horizontal"=w141:i32, "Vertical"=w134:i32)
        n337 = property on="Curves Tree" class="Tree (strict)"() -> ("Height"=w143:u32, "Width"=w144:u32, "Left"=w142:i32, "Top"=w135:i32)  [unwired: 2 in, 2 out]
        n338 = Add(x=w144, y=w142) -> (x+y=w140:u32)
        n339 = Add(x=w143, y=w135) -> (x+y=w133:u32)
        n340 = Less?(x=w141, y=w142) -> (x < y?=w138:bool)
        n341 = Greater?(x=w141, y=w140) -> (0:w139:bool)
        n342 = Less?(x=w134, y=w135) -> (x < y?=w137:bool)
        n343 = Greater?(x=w134, y=w133) -> (0:w136:bool)
        n344 = Or(x=w138, y=w139) -> (x .or. y?=w132:bool)
        n345 = Or(x=w137, y=w136) -> (x .or. y?=w131:bool)
        n346 = Or(x=w132, y=w131) -> (x .or. y?=w130:bool)
        n347 = case shown="True" w130 {
          frame False {
          }
          frame True {
            n348 = local write "DragStartFlag"(FALSE ("DragStartFlag")) -> ()
            n349 = property on="BottomBar" class="Bool (strict)"("Visible"=FALSE) -> ()  [unwired: 2 in, 2 out]
          }
        }
      }
      frame Default {
      }
    }
    n350 = Unbundle By Name(w94) -> ("Width"=w93:bool, "Height"=w92:bool)
    n351 = Or(x=w93, y=w92) -> (x .or. y?=w91:bool)
    n352 = case shown="True" w91 {
      tunnel: w90 -> [_ w110]
      frame False {
      }
      frame True {
        n353 = control-ref of="Splitter"() -> (w108:refnum<vi>)
        n354 = local write "OldPos"(w110) -> ()
        n355 = control-ref of="Pane"() -> (w109:refnum<vi>)
        n356 = control-ref of="Pane 2"() -> (w107:refnum<vi>)
        n357 = call "CRYInit Listbox.vi"("Pane 2"=w107, "Splitter"=w108, "Pane 1"=w109) -> ()  [unwired: 9 in]
      }
    }
    n358 = local write "DragStartFlag"(FALSE ("DragStartFlag")) -> ()
    n359 = property on="BottomBar" class="Bool (strict)"("Visible"=FALSE) -> ()  [unwired: 2 in, 2 out]
    n360 = case shown="2..5" w102 {
      frame Default {
      }
      frame 2..5 {
        n361 = call "CRYUpdate Buttons.vi"() -> ()  [unwired: 1 in, 11 out]
      }
    }
  }
  n362 = while {
    tunnel: w7 -> [w548]
    tunnel: [w549] -> w9
    shift-right: [w543] -> w5
    shift-left: w6 -> [w546]
    stop <- w549 stop-if-true
    n363 = Get Queue Status(queue=w548, error in (no error)=w546) -> (queue out=w547:refnum<queue>, error out=w543:errorcluster, # elements in queue=w544:i32)  [unwired: 6 out]
    n364 = Wait (ms)(milliseconds to wait=u32 10) -> ()  [unwired: 1 out]
    n365 = case shown="Default" w544 {
      tunnel: w547 -> [_ w556]
      tunnel: w543 -> [_ w555]
      frame 0 {
        n366 = Wait (ms)(milliseconds to wait=u32 10) -> ()  [unwired: 1 out]
      }
      frame Default {
        n367 = Dequeue Element(queue=w556, error in (no error)=w555) -> (element=w553:string, error out=w554:errorcluster)  [unwired: 3 out]
        n368 = case shown="No Error" w554 {
          tunnel: w553 -> [w560 _]
          frame No Error {
            n369 = Scan From String(format string="%s%s%d%d", input string=w560) -> (output 1=w558:string, output 2=w557:string, output 3=w559:i32)  [unwired: 2 in, 8 out]
            n370 = case shown="\"Mouse_Down\"" w558 {
              selector: w558 -> [_ w562 _ w594]
              tunnel: w559 -> [_ w564 w566 w597]
              tunnel: w557 -> [_ _ w570 w596]
              frame Default {
              }
              frame "Mouse_Down" {
                n371 = local read "Coords"() -> (w565:T1)
                n372 = To Unsigned Word Integer(number=w564) -> (unsigned 16bit integer=w563:u16)
                n373 = call "CRYCurve Library Interface.vi"("nButton"=w563, "Coords"=w565, "sEventName"=w562) -> ()  [unwired: 8 in, 1 out]
              }
              frame "Intensity_Insert" {
                n374 = Concatenate Strings(w570, "&" ("string"), "INTENSITY" ("GraphType")) -> (w567:string)
                n375 = call "CRYGraph View Socket Client.vi"("sOption"="BELOW_INSERT", "nData"=w566, "sData"=w567, "sAction"="GET_GRAPHWINDOW") -> ("bResult Out"=w572:bool, "pVI Out"=w571:refnum<vi>)  [unwired: 4 in, 2 out]
                n376 = case shown="True" w572 {
                  tunnel: w571 -> [_ w591]
                  tunnel: w566 -> [_ w593]
                  tunnel: w570 -> [_ w592]
                  frame False {
                  }
                  frame True {
                    n377 = call "CRYGraph View Socket Client.vi"("sOption"="FROM_GRAPHNUMBER", "nData"=w593, "sData"=w592, "sAction"="GET_GRAPHWINDOW") -> ("pVI Out"=w576:refnum<vi>)  [unwired: 4 in, 3 out]
                    n378 = call "CRYGet Graph Window Information.vi"("pGraph VI In"=w576) -> ("Legend Ref Out"=w575:refnum<vi>)  [unwired: 4 in, 10 out]
                    n379 = call "CRYGet Graph Data in Graph.vi"("Graph Type"="WAVE", "Legend Refnum"=w575, "Type In"=enum16{"Curves", "Values", "Results", "WFM"}."WFM") -> ("Rows"=w585:i32[])  [unwired: 4 in, 4 out]
                    n380 = Index Array(array=w585) -> (element=w584:i32)  [unwired: 1 in]
                    n381 = Build Array(w584) -> (w583:i32[])
                    n382 = call "CRYPlot Intensity Graph.vi"("pGraph VI In"=w591, "Selected Rows In"=w583) -> ("ItemSyms"=w588:i32[], "Color Info"=w590:u32[], "Wave Names"=w589:string[], "All Rows Out"=w582:i32[])  [unwired: 6 in]
                    n383 = call "CRYData View Legend New Insert.vi"("Item Symbols"=w588, "Color Array"=w590, "ItemName Array"=w589, "pGraph VI In"=w591) -> ()  [unwired: 1 in, 7 out]
                    n384 = call "CRYGet Current CurLib Listbox.vi"() -> ("Type"=w581:enum16{"Curves", "Values", "Results", "WFM"})  [unwired: 9 in, 2 out]
                    n385 = call "CRYSymbol Conversion.vi"("CurLib Tab Type"=w581, "nDatas"=w582, "sData"="TAB_CHANGE" ("sActin"), "sActin"="ACTIVE") -> ()  [unwired: 8 in]
                  }
                }
              }
              frame "POLAR_XY" {
                n386 = call "CRYGraph View Socket Client.vi"("sOption"="FROM_GRAPHNUMBER", "nData"=w597, "sData"=w596, "sAction"="GET_GRAPHWINDOW") -> ("pVI Out"=w595:refnum<vi>)  [unwired: 4 in, 3 out]
                n387 = call "CRYGraph Property Window Main.vi"("TabName"=w594, "pGraph VI In"=w595) -> ()  [unwired: 1 in, 9 out]
              }
            }
          }
          frame Error {
          }
        }
      }
    }
    n388 = Unbundle By Name(w543) -> ("status"=w550:bool)
    n389 = local read "stop"() -> (w551:bool)
    n390 = Or(x=w551, y=w550) -> (x .or. y?=w549:bool)
  }
  n391 = Release Queue(queue=w7, error in (no error)=w5) -> (error out=w8:errorcluster)  [unwired: 3 out]
  n392 = flat-sequence {
    tunnel: w8 -> [w601]
    tunnel: w9 -> [w602]
    tunnel: w12 -> [w603]
    tunnel: [w603] -> w16
    tunnel: [w602] -> w15
    tunnel: [w601] -> w14
    tunnel: w16 -> [_]
    tunnel: w15 -> [_]
    tunnel: w14 -> [_]
    frame #0 {
      n393 = call "CRYProbe Window Close.vi"() -> ()  [unwired: 1 in]
      n394 = property on="BottomBar" class="Bool (strict)"("Visible"=FALSE) -> ()  [unwired: 2 in, 2 out]
    }
    frame #1 {
      n395 = global write "CRYCurve Library Global.vi" "Curve Library Exist"(FALSE ("Curve Library Exist")) -> ()
      n396 = local write "StateOut"(TRUE ("StateOut")) -> ()
    }
  }
  n397 = call-poly <vilib>:"Close Input Device.vi"("error in (no error)"=w1, "device ID"=w2) -> ()  [unwired: 8 in, 1 out]
